vi "Sample--Sync_BackplaneRefClk_PXI.vi"() -> ()   [LabVIEW 2013]
doc: "This example demonstrates synchronizing two digitizers."
uses:
  <userlib>/ArtScope/Trigger/ArtScope_ConfigureTriggerDigital.vi
  <userlib>/ArtScope/Fetch/ArtScope_FetchBinary16.vi
  <userlib>/ArtScope/_SubVI/ArtScope_ArrayByChannel_U16.vi
panel:
  out "error out":errorcluster
  in  "reference position2":dbl
  in  "reference position":dbl
  out "Data 2":u16[][](graph)
  in  "range(Vpp)":i32(ring) items=["20V", "10V", "2V", "40V", "16V", "8V", "4V", "1.6V", "800m", "400m", "160m", "80m", "40m"]
  in  "range(Vpp)":i32(ring) items=["20V", "10V", "2V", "40V", "16V", "8V", "4V", "1.6V", "800m", "400m", "160m", "80m", "40m"]
  in  "Slave":string="Dev2"
  in  "Master":string="Dev1"
  in  "Stop":bool
  in  "Timeout(s) 2":dbl=1.0
  in  "MinSampleRate 2":dbl=8000000.0
  in  "MinRecordLength2":i32=6000
  out "Data":u16[][](graph)
  in  "Timeout(s)":dbl=1.0
  in  "MinRecordLength":i32=6000
  in  "MinSampleRate":dbl=8000000.0
  # "Vertical"
  # "Horizontal"
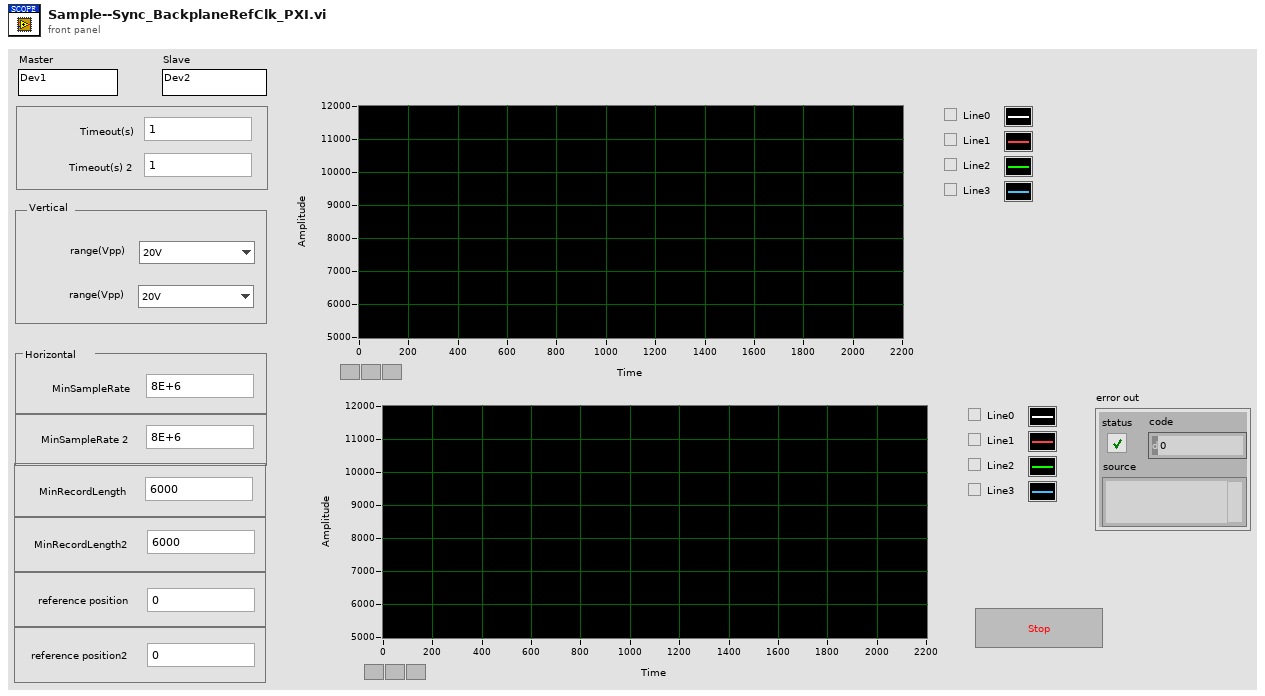
[diagram p1: front panel]
types:
  T1 = cluster{"fLSB":cluster{dbl, dbl, dbl, dbl, dbl, dbl, dbl, dbl}, "RangeValue":cluster{dbl, dbl, dbl, dbl, dbl, dbl, dbl, dbl}, "wMaxLSB":u32, "TriggerMode":i32, "sampLengthPerChan":u32, "pAvailSampsPoints":u32, "channelCount":i32}
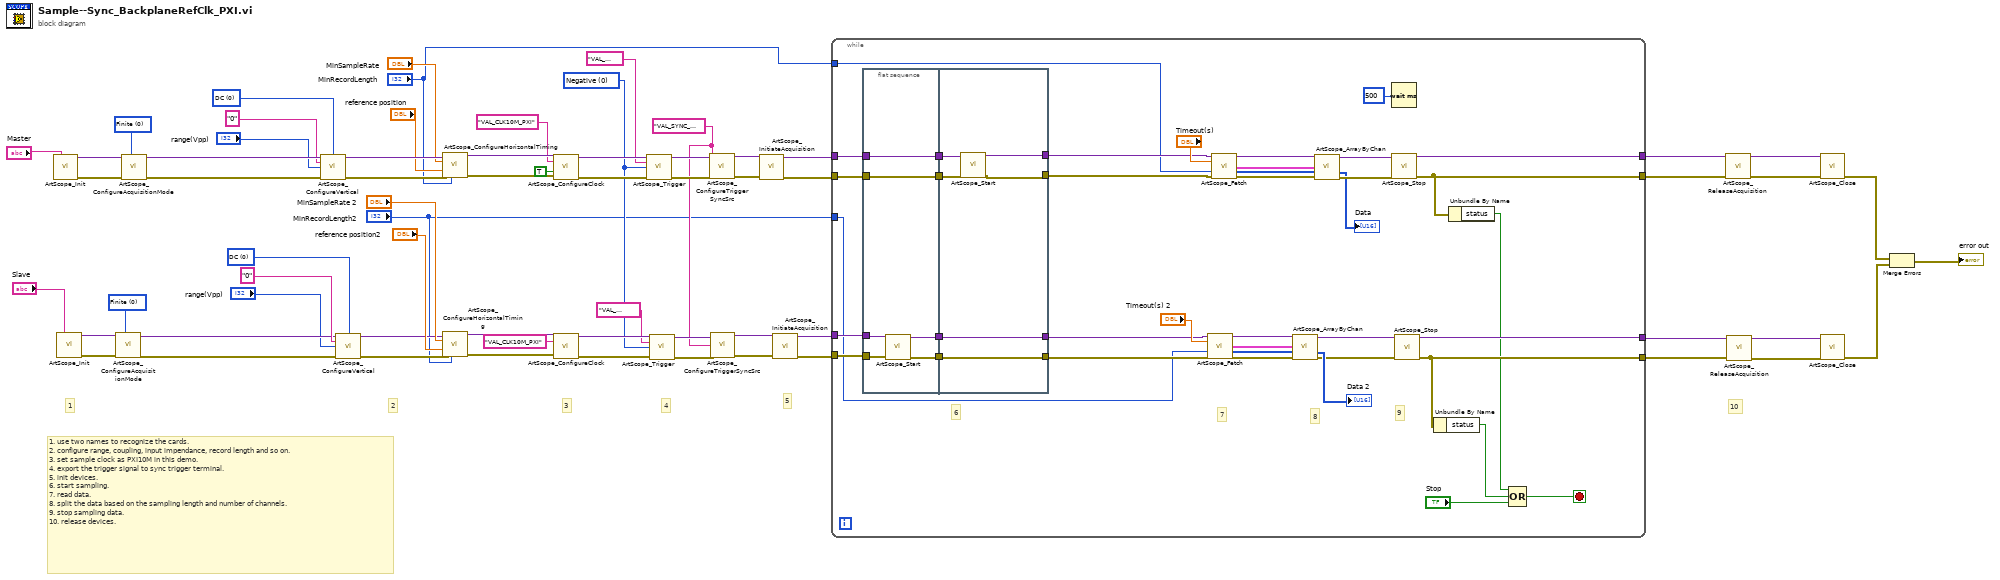
[diagram p0: block diagram]
diagram:
  w6 = "VAL_SYNC_TRIGGER0" ("trigger sync source")
  w15 = 0 items=["Negative", "Positive", "NegatPosit"] ("edge")
  w46 = 0 items=["DC", "AC"] ("Coupling")
  w54 = 0 items=["Finite", "Continuous"] ("AcuqMode")
  w64 = 0 items=["DC", "AC"] ("Coupling")
  w59 = 0 items=["Finite", "Continuous"] ("AcuqMode")
  # "1. use two names to recognize the cards.\n2. configure range, coupling, input impendance, record length and so on.\n3. set sample clock as PXI10M in this demo.\n4. export the trigger signal to sync trigger terminal.\n5. init devices.\n6. start sampling.\n7. read data.\n8. split the data based on the sampling length and number of channels.\n9. stop sampling data.\n10. release devices."
  # "10"
  # "5"
  # "4"
  # "3"
  # "2"
  # "1"
  n1 = call <userlib>:"ArtScope_Init.vi"("task name"="Master") -> ("task handle"=w42:variant, "error out"=w41:errorcluster)  [unwired: 13 in]
  n2 = call <userlib>:"ArtScope_Init.vi"("task name"="Slave") -> ("task handle"=w39:variant, "error out"=w38:errorcluster)  [unwired: 13 in]
  n3 = call <userlib>:"ArtScope_ConfigureAcquisitionMode.vi"("task handle"=w39, "acquisition mode"=w54, "error in (no error)"=w38) -> ("task handle"=w45:variant, "error out"=w44:errorcluster)  [unwired: 11 in]
  n4 = call <userlib>:"ArtScope_ConfigureAcquisitionMode.vi"("task handle"=w42, "acquisition mode"=w59, "error in (no error)"=w41) -> ("task handle"=w58:variant, "error out"=w60:errorcluster)  [unwired: 11 in]
  n5 = call <userlib>:"ArtScope_ConfigureVertical.vi"("task handle"=w58, "coupling"=w64, "channels"="0" ("Channel Name"), "range(Vpp)"="range(Vpp)", "error in (no error)"=w60) -> ("task handle"=w63:variant, "error out"=w62:errorcluster)  [unwired: 9 in]
  n6 = call <userlib>:"ArtScope_ConfigureVertical.vi"("task handle"=w45, "coupling"=w46, "channels"="0" ("Channel Name"), "range(Vpp)"="range(Vpp)", "error in (no error)"=w44) -> ("task handle"=w47:variant, "error out"=w48:errorcluster)  [unwired: 9 in]
  n7 = call <userlib>:"ArtScope_ConfigureHorizontalTiming.vi"("task handle"=w63, "min sample rate"="MinSampleRate", "reference position"="reference position", "error in (no error)"=w62, "min record length"="MinRecordLength") -> ("task handle"=w43:variant, "error out"=w57:errorcluster)  [unwired: 9 in]
  n8 = call <userlib>:"ArtScope_ConfigureHorizontalTiming.vi"("task handle"=w47, "min sample rate"="MinSampleRate 2", "reference position"="reference position2", "error in (no error)"=w48, "min record length"="MinRecordLength2") -> ("task handle"=w51:variant, "error out"=w50:errorcluster)  [unwired: 9 in]
  n9 = call <userlib>:"ArtScope_ConfigureClock.vi"("task handle"=w43, "input clock source"="VAL_CLK10M_PXI", "master enable"=TRUE, "error in (no error)"=w57) -> ("task handle"=w21:variant, "error out"=w20:errorcluster)  [unwired: 10 in]
  n10 = call <userlib>:"ArtScope_ConfigureClock.vi"("task handle"=w51, "input clock source"="VAL_CLK10M_PXI", "error in (no error)"=w50) -> ("task handle"=w18:variant, "error out"=w17:errorcluster)  [unwired: 11 in]
  n11 = call-poly <userlib>:"ArtScope_Trigger.vi"("task handle"=w21, "trigger source"="VAL_TRIGGER_DTR", "edge"=w15, "error in"=w20) -> ("task handle"=w11:variant, "error out"=w14:errorcluster)  [unwired: 10 in]
  n12 = call-poly <userlib>:"ArtScope_Trigger.vi"("task handle"=w18, "trigger source"="VAL_TRIGGER_SYNCTRIGGER", "edge"=w15, "error in"=w17) -> ("task handle"=w10:variant, "error out"=w8:errorcluster)  [unwired: 10 in]
  n13 = call <userlib>:"ArtScope_ConfigureTriggerSyncSrc.vi"("task handle"=w11, "trigger sync source"=w6, "error in (no error)"=w14) -> ("task handle"=w12:variant, "error out"=w13:errorcluster)  [unwired: 11 in]
  n14 = call <userlib>:"ArtScope_ConfigureTriggerSyncSrc.vi"("task handle"=w10, "trigger sync source"=w6, "error in (no error)"=w8) -> ("task handle"=w9:variant, "error out"=w7:errorcluster)  [unwired: 11 in]
  n15 = call <userlib>:"ArtScope_InitiateAcquisition.vi"("task handle"=w12, "error in (no error)"=w13) -> ("task handle"=w33:variant, "error out"=w34:errorcluster)  [unwired: 12 in]
  n16 = call <userlib>:"ArtScope_InitiateAcquisition.vi"("task handle"=w9, "error in (no error)"=w7) -> ("task handle"=w36:variant, "error out"=w35:errorcluster)  [unwired: 12 in]
  n17 = while {
    tunnel: [w103] -> w32
    tunnel: [w90] -> w30
    tunnel: [w92] -> w28
    tunnel: [w102] -> w25
    tunnel: w36 -> [w101]
    tunnel: w35 -> [w100]
    tunnel: w33 -> [w96]
    tunnel: w34 -> [w95]
    tunnel: "MinRecordLength" -> [w82]
    tunnel: "MinRecordLength2" -> [w81]
    stop <- w87 stop-if-true
    # "9"
    # "8"
    # "7"
    # "6"
    n18 = flat-sequence {
      tunnel: w101 -> [w111]
      tunnel: w100 -> [w110]
      tunnel: [w106] -> w105
      tunnel: [w109] -> w104
      tunnel: [w108] -> w97
      tunnel: w96 -> [w108]
      tunnel: w95 -> [w107]
      tunnel: [w107] -> w94
      tunnel: w105 -> [w117]
      tunnel: w104 -> [w116]
      tunnel: w97 -> [w115]
      tunnel: w94 -> [w114]
      tunnel: [w112] -> w85
      tunnel: [w113] -> w86
      tunnel: [w117] -> w84
      tunnel: [w116] -> w83
      frame #0 {
        n19 = call <userlib>:"ArtScope_Start.vi"("task handle"=w111, "error in (no error)"=w110) -> ("task handle"=w106:variant, "error out"=w109:errorcluster)  [unwired: 12 in]
      }
      frame #1 {
        n20 = call <userlib>:"ArtScope_Start.vi"("task handle"=w115, "error in (no error)"=w114) -> ("task handle"=w113:variant, "error out"=w112:errorcluster)  [unwired: 12 in]
      }
    }
    n21 = call-poly <userlib>:"ArtScope_Fetch.vi"("task handle"=w84, "timeout"="Timeout(s) 2", "num samples"=w81, "error in (no error)"=w83) -> ("task handle"=w73:variant, "wfm info"=w71:T1, "data"=w70:u16[], "error out"=w72:errorcluster)  [unwired: 8 in]
    n22 = call-poly <userlib>:"ArtScope_Fetch.vi"("task handle"=w86, "timeout"="Timeout(s)", "num samples"=w82, "error in (no error)"=w85) -> ("task handle"=w79:variant, "wfm info"=w76:T1, "data"=w75:u16[], "error out"=w80:errorcluster)  [unwired: 8 in]
    n23 = call-poly <userlib>:"ArtScope_ArrayByChan.vi"("task handle"=w73, "wfm info"=w71, "1D data"=w70, "error in (no error)"=w72) -> ("task handle"=w69:variant, "2D data"=→"Data 2":u16[][], "error out"=w67:errorcluster)  [unwired: 9 in]
    n24 = call-poly <userlib>:"ArtScope_ArrayByChan.vi"("task handle"=w79, "wfm info"=w76, "1D data"=w75, "error in (no error)"=w80) -> ("task handle"=w78:variant, "2D data"=→"Data":u16[][], "error out"=w77:errorcluster)  [unwired: 9 in]
    n25 = call <userlib>:"ArtScope_Stop.vi"("task handle"=w78, "error in"=w77) -> ("task handle"=w103:variant, "error out"=w90:errorcluster)  [unwired: 12 in]
    n26 = Wait (ms)(milliseconds to wait=u32 500 ("等待时间（毫秒）")) -> ()  [unwired: 1 out]
    n27 = call <userlib>:"ArtScope_Stop.vi"("task handle"=w69, "error in"=w67) -> ("task handle"=w102:variant, "error out"=w92:errorcluster)  [unwired: 12 in]
    n28 = Unbundle By Name(w92) -> ("status"=w91:bool)
    n29 = Unbundle By Name(w90) -> ("status"=w89:bool)
    n30 = Compound Arithmetic op=OR(w89, w91, "Stop") -> (w87:bool)
  }
  n31 = call <userlib>:"ArtScope_ReleaseAcquisition.vi"("task handle"=w32, "error in (no error)"=w30) -> ("task handle"=w31:variant, "error out"=w29:errorcluster)  [unwired: 12 in]
  n32 = call <userlib>:"ArtScope_ReleaseAcquisition.vi"("task handle"=w25, "error in (no error)"=w28) -> ("task handle"=w26:variant, "error out"=w27:errorcluster)  [unwired: 12 in]
  n33 = call <userlib>:"ArtScope_Close.vi"("task handle"=w31, "error in (no error)"=w29) -> ("error out"=w66:errorcluster)  [unwired: 13 in]
  n34 = call <userlib>:"ArtScope_Close.vi"("task handle"=w26, "error in (no error)"=w27) -> ("error out"=w65:errorcluster)  [unwired: 13 in]
  n35 = Merge Errors(w66, w65) -> (→"error out":errorcluster)
